vi "Export Origin - cDLTS.vi"(8 "Error In":errorcluster, 9 "Workspace":path, 10 "Session properties":T2, 11 "cDLTS measurement":T3={"Name"="", "Comment"="", "Time"=timestamp(0 s since 1904-01-01), "Folder"=path "", "DLTS properties"={"Tstart"=100.0, "Instant start"=FALSE, "Tstop"=350.0, "T rate"=0.016666666666666666, "Test signal"=0.1, "Test frequency"=100000.0, "Bandwidth"=0.0, "Averaging"=5.0, "Vbias"=-5.0, "Vpulse"=-1.0, "pulse length"=0.1, "Pulse 2"=FALSE, "Vpulse 2"=0.0, "pulse length 2"=0.0, "I range"=-2.0, "V range"=10.0, "Emission rate"=[10.0], "Sampling rate"=107000.0, "Acq. delay"=0.0}, "GUID"=""} {"DLTS properties"."V range" items=["10mV"=0.01, "100mV"=0.1, "1V"=1.0, "10V"=10.0]; "DLTS properties"."I range" items=["10mV"=0.01, "100mV"=0.1, "1V"=1.0, "10V"=10.0]}) -> (0 "Error Out":errorcluster)   [LabVIEW 2019]
doc: "Handles export of a DLTS measurement to an Origin project, displays a GUI window"
uses:
  Type defs/cDLTS measurement Type Def.ctl
  Type defs/DLTS properties Type Def.ctl
  Type defs/Session properties Type Def.ctl
  <vilib>/Utility/sysdir.llb/System Directory Type.ctl
panel:
  in  "Comment":T1(array[ring])=[enum."Emission rate"] caption="Parameters to be placed in comments"
  in  "Save and exit after export":bool
  in  "Export to current Origin instance":bool
  out "String":string
  in  "Path":path caption="Export file as:"
  in  "Export":bool
  in  "Cancel":bool
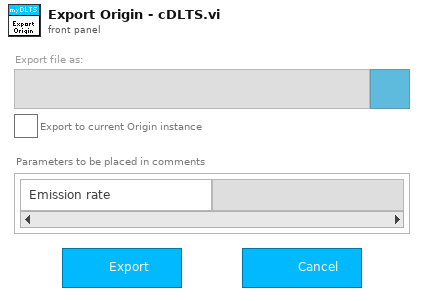
[diagram p1: front panel]
types:
  T1 = enum16{"", "Emission rate", "Temperature change rate", "Test signal", "Test frequency", "Bandwidth", "Averaging", "Bias voltage", "Pulse 1 voltage", "Pulse 1 length", "Pulse 2 voltage", "Pulse 2 length", "Current range", "Voltage range", "Sampling rate", "Acquisition delay"}[]
  T2 = typedef "Session properties Type Def.ctl" = cluster{"Session name":string, "Comment":string, "User":string, "Software version":dbl, "Created":timestamp, "Modified":timestamp, "Binary":bool, "GUID":string}
  T3 = typedef "cDLTS measurement Type Def.ctl" = cluster{"Name":string, "Comment":string, "Time":timestamp, "Folder":path, "DLTS properties":T4, "GUID":string}
  T4 = typedef "DLTS properties Type Def.ctl" = cluster{"Tstart":dbl[unit], "Instant start":bool, "Tstop":dbl[unit], "T rate":dbl[unit], "Test signal":dbl[unit], "Test frequency":dbl[unit], "Bandwidth":dbl[unit], "Averaging":dbl, "Vbias":dbl[unit], "Vpulse":dbl[unit], "pulse length":dbl[unit], "Pulse 2":bool, "Vpulse 2":dbl[unit], "pulse length 2":dbl[unit], "I range":dbl, "V range":dbl[unit], "Emission rate":dbl[unit][], "Sampling rate":dbl[unit], "Acq. delay":dbl[unit]}
  T5 = enum32{"existing file", "new file", "new or existing file", "existing dir", "new dir", "new or existing dir", "existing file (use LLBs)", "new file (use LLBs)", "new or existing file (use LLBs)", "new or existing file or directory (use LLBs)", "existing dir (use LLBs)", "new dir (use LLBs)", "new or existing dir (use LLBs)", "existing file or dir", "new file or dir", "new or existing file or dir", "existing file or dir (use LLBs)", "new file or dir (use LLBs)"}
  T6 = typedef "System Directory Type.ctl" = i32
  T7 = enum8{"Enabled", "Disabled", "Disabled and Grayed Out"}
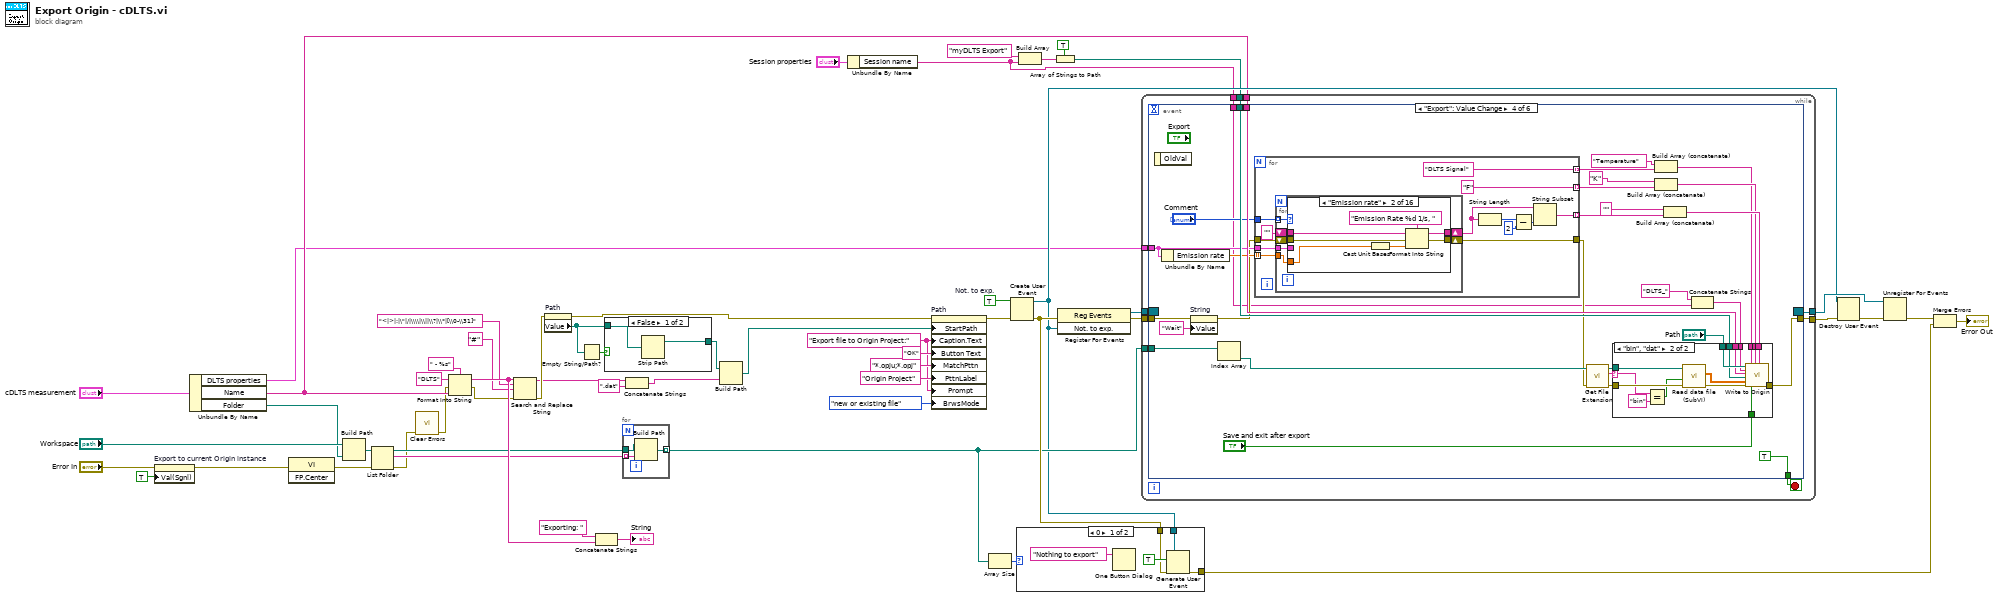
[diagram p0: block diagram]
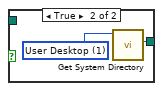
[diagram p2: hidden frame]
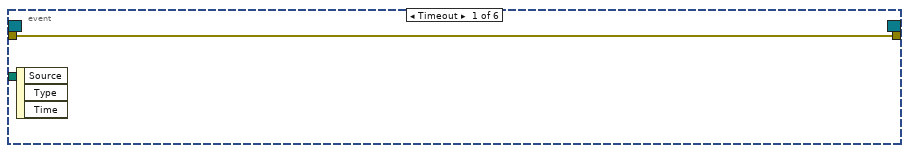
[diagram p4: hidden frame]
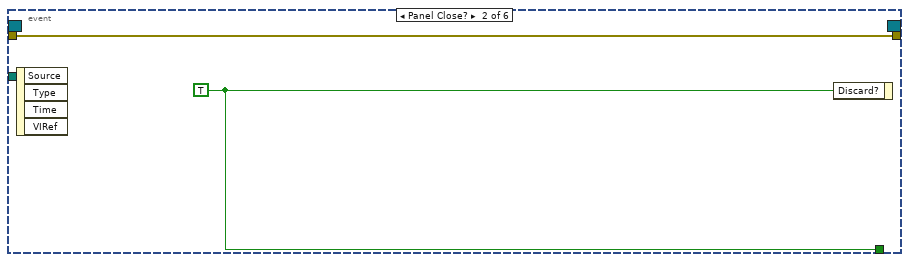
[diagram p5: hidden frame]
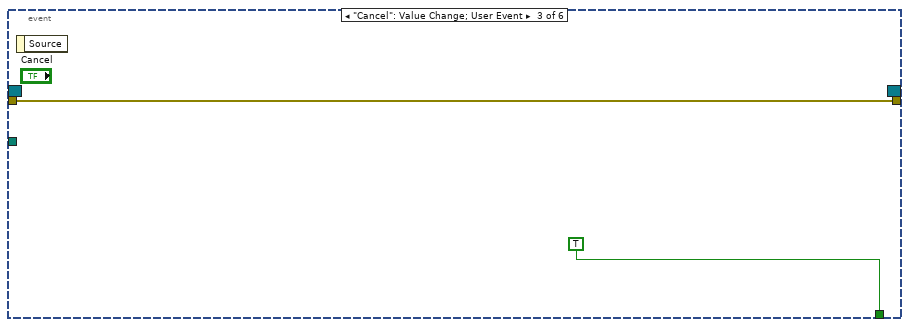
[diagram p6: hidden frame]
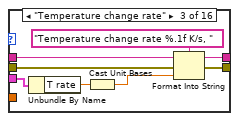
[diagram p8: hidden frame]
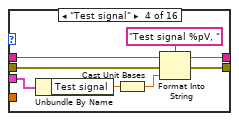
[diagram p9: hidden frame]
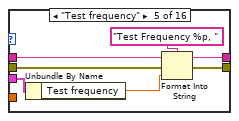
[diagram p10: hidden frame]
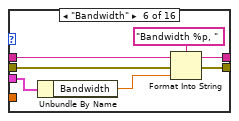
[diagram p11: hidden frame]
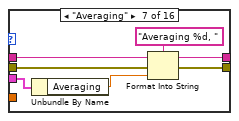
[diagram p12: hidden frame]
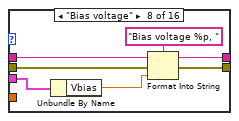
[diagram p13: hidden frame]
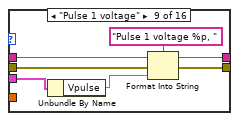
[diagram p14: hidden frame]
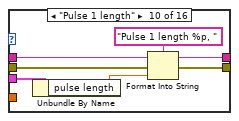
[diagram p15: hidden frame]
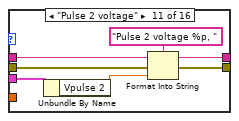
[diagram p16: hidden frame]
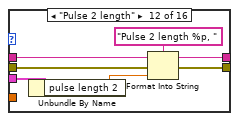
[diagram p17: hidden frame]
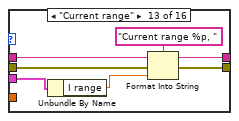
[diagram p18: hidden frame]
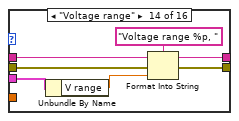
[diagram p19: hidden frame]
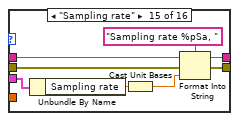
[diagram p20: hidden frame]
diagram:
  w27 = "Export file to Origin Project:"
  w54 = TRUE  # Not. to exp.
  n1 = property on="Export to current Origin instance" class="Bool (strict)"(error in="Error In", "Val(Sgnl)"=TRUE ("Value (Signaling)")) -> (error out=w6:errorcluster)  [unwired: 1 in, 1 out]
  n2 = Unbundle By Name("cDLTS measurement") -> ("DLTS properties"=w3:T4, "Name"=w14:string, "Folder"=w32:path)
  n3 = invoke class="VI" method="FP.Center"(error in=w6) -> (error out=w16:errorcluster)  [unwired: 2 in, 2 out]
  n4 = Build Path(base path="Workspace", name or relative path=w32) -> (appended path=w25:path)
  n5 = List Folder(path=w25, error in=w16) -> (path out=w24:path, filenames=w31:string[], error out=w20:errorcluster)  [unwired: 2 in, 1 out]
  n6 = call <vilib>:"Clear Errors.vi"("error in (no error)"=w20) -> ("error out"=w1:errorcluster)  [unwired: 5 in, 1 out]
  n7 = Format Into String(format string=" - %s", initial string="DLTS", error in=w1, w14) -> (resulting string=w43:string, error out=w19:errorcluster)
  n8 = Search and Replace String(input string=w43, search string="<|>|:|\"|/|\\\\|\\||\\?|\\*|[\\0-\\31]", replace string="#" ("replace string (\"\")"), error in=w19) -> (result string=w18:string, error out=w21:errorcluster)  [unwired: 4 in, 2 out]
  n9 = property on="Path" class="Path"(error in=w21) -> (error out=w33:errorcluster, "Value"=w39:path)  [unwired: 1 in, 1 out]
  n10 = Empty String/Path?(string/path=w39) -> (empty?=w40:bool)
  n11 = Concatenate Strings("Exporting: " ("string"), w43) -> (→"String":string)
  n12 = case shown="False" w40 {
    tunnel: w39 -> [w58 _]
    tunnel: [w57 w59] -> w35
    frame False {
      n13 = Strip Path(path=w58) -> (stripped path=w57:path)  [unwired: 1 out]
    }
    frame True {
      w60 = T6 1 items=["User Home"=0, "User Desktop"=1, "User Documents"=2, "User Application Data"=3, "User Preferences"=4, "User Temporary"=5, "Public Documents"=6, "Public Application Data"=7, "Public Preferences"=8, "Public Cache"=13, "System Core Libraries"=9, "System Installed Libraries"=10, "Application Files"=11, "Boot Volume Root"=12] ("system directory type")
      n14 = call <vilib>:"Get System Directory.vi"("system directory type"=w60) -> ("system directory"=w59:path)  [unwired: 10 in]
    }
  }
  n15 = for {
    tunnel: w24 -> [w63]
    tunnel: [w62] -> w49 mode=indexing
    tunnel: w31 -> [w61] mode=indexing
    n16 = Build Path(base path=w63, name or relative path=w61) -> (appended path=w62:path)
  }
  n17 = Concatenate Strings(w18, ".dat" ("string")) -> (w22:string)
  n18 = Build Path(base path=w35, name or relative path=w22) -> (appended path=w34:path)
  n19 = Unbundle By Name("Session properties") -> ("Session name"=w2:string)
  n20 = property on="Path" class="Path"(error in=w33, "StartPath"=w34, "Caption.Text"=w27, "Button Text"="OK", "MatchPttn"="*.opju;*.opj", "PttnLabel"="Origin Project", "Prompt"=w27, "BrwsMode"=T5."new or existing file" ("Browse Options:Selection Mode")) -> (error out=w51:errorcluster)  [unwired: 1 in, 1 out]
  n21 = Array Size(array=w49) -> (size(s)=w55:i32)
  n22 = Create User Event(user event datatype=w54, error in=w51) -> (user event=w15:refnum<user-event>, error out=w50:errorcluster)
  n23 = case shown="0" w55 {
    tunnel: w15 -> [w67 _]
    tunnel: w50 -> [w65 w69]
    tunnel: [w64 w69] -> w44
    frame 0 {
      n24 = One Button Dialog(message="Nothing to export") -> ()  [unwired: 1 in, 1 out]
      n25 = Generate User Event(user event=w67, event data cluster=TRUE ("event data"), error in=w65) -> (error out=w64:errorcluster)  [unwired: 1 in, 1 out]
    }
    frame Default {
    }
  }
  n26 = Build Array("myDLTS Export" ("element"), w2) -> (w10:string[])
  n27 = Array of Strings to Path(0:w10, 1:TRUE ("relative")) -> (2:w9:path)
  n28 = register-events(error in=w50, w15) -> (reference out=w52:refnum<event-registration>, error out=w53:errorcluster)  [unwired: 1 in]
  n29 = while {
    tunnel: w53 -> [w79]
    tunnel: w49 -> [w77]
    tunnel: w52 -> [w76]
    tunnel: [w75] -> w47
    tunnel: w14 -> [w74]
    tunnel: w9 -> [w73]
    tunnel: [w72] -> w8
    tunnel: w3 -> [w71]
    tunnel: w2 -> [w70]
    stop <- w78 stop-if-true
    n30 = event shown="[3] \"Export\": Value Change" {
      selector: w76 -> [_ _ _ _ _ _]
      dyn-events: [_ _ _ _ _ _] -> w75
      timeout: _ -> [_ _ _ _ _ _]
      tunnel: w79 -> [w80 w81 w83 w109 w269 w276]
      tunnel: [w80 w81 w83 w112 w262 w271] -> w72
      tunnel: [_ w82 TRUE ("Discard?") TRUE _ _] -> w78
      tunnel: w77 -> [_ _ _ w114 _ _]
      tunnel: w74 -> [_ _ _ w107 _ _]
      tunnel: w73 -> [_ _ _ w106 _ _]
      tunnel: w71 -> [_ _ _ w90 _ _]
      tunnel: w70 -> [_ _ _ w85 _ _]
      event Timeout {
        n31 = event-data() -> ()  [unwired: 1 in, 3 out]
      }
      event Panel Close? {
        w82 = TRUE ("Discard?")
        n32 = event-data() -> ()  [unwired: 1 in, 4 out]
        n33 = event-data("Discard?"=w82) -> ()  [unwired: 1 in, 1 out]
      }
      event "Cancel": Value Change; User Event {
        n34 = event-data() -> ()  [unwired: 1 in, 1 out]
      }
      event "Export": Value Change {
        n35 = event-data() -> ()  [unwired: 1 in, 1 out]
        n36 = Unbundle By Name(w90) -> ("Emission rate"=w91:dbl[unit][])
        n37 = property on="String" class="Str"(error in=w109, "Value"="Wait" ("String")) -> (error out=w89:errorcluster)  [unwired: 1 in, 1 out]
        n38 = Index Array(array=w114) -> (element=w102:path)  [unwired: 1 in]
        n39 = for {
          tunnel: w90 -> [w123]
          tunnel: [w119] -> w98 mode=indexing
          tunnel: ["DLTS Signal"] -> w100 mode=indexing
          tunnel: ["F"] -> w99 mode=indexing
          tunnel: "Comment" -> [w125]
          tunnel: w91 -> [w122] mode=indexing
          tunnel: w89 -> [w121]
          tunnel: [w120] -> w88
          n40 = for {
            tunnel: w125 -> [w134] mode=indexing
            tunnel: w123 -> [w133]
            shift-right: [w132] -> w120
            shift-left: w121 -> [w131]
            shift-right: [w130] -> w118
            shift-left: "" -> [w129]
            tunnel: w122 -> [w128]
            n41 = case shown="\"Emission rate\"" w134 {
              tunnel: w133 -> [_ _ w147 w153 w160 w167 w174 w181 w188 w195 w202 w209 w216 w223 w231 w238]
              tunnel: w128 -> [_ w142 _ _ _ _ _ _ _ _ _ _ _ _ _ _]
              tunnel: [w135 w141 w151 w157 w162 w171 w178 w185 w192 w199 w206 w213 w220 w227 w235 w242] -> w132
              tunnel: w131 -> [w135 w140 w149 w155 w164 w169 w176 w182 w189 w196 w203 w210 w217 w224 w232 w239]
              tunnel: [w136 w139 w150 w156 w161 w170 w177 w184 w191 w198 w205 w212 w219 w226 w234 w241] -> w130
              tunnel: w129 -> [w136 w138 w148 w154 w163 w168 w175 w183 w190 w197 w204 w211 w218 w225 w233 w240]
              frame "", Default {
              }
              frame "Emission rate" {
                n42 = Cast Unit Bases(0:w142) -> (2:w137:dbl)  [unwired: 1 in]
                n43 = Format Into String(format string="Emission Rate %d 1/s, ", initial string=w138, error in=w140, w137) -> (resulting string=w139:string, error out=w141:errorcluster)
              }
              frame "Temperature change rate" {
                n44 = Unbundle By Name(w147) -> ("T rate"=w146:dbl[unit])
                n45 = Cast Unit Bases(0:w146) -> (2:w144:dbl)  [unwired: 1 in]
                n46 = Format Into String(format string="Temperature change rate %.1f K/s, ", initial string=w148, error in=w149, w144) -> (resulting string=w150:string, error out=w151:errorcluster)
              }
              frame "Test signal" {
                n47 = Unbundle By Name(w153) -> ("Test signal"=w158:dbl[unit])
                n48 = Cast Unit Bases(0:w158) -> (2:w152:dbl)  [unwired: 1 in]
                n49 = Format Into String(format string="Test signal %pV, ", initial string=w154, error in=w155, w152) -> (resulting string=w156:string, error out=w157:errorcluster)
              }
              frame "Test frequency" {
                n50 = Unbundle By Name(w160) -> ("Test frequency"=w165:dbl[unit])
                n51 = Format Into String(format string="Test Frequency %p, ", initial string=w163, error in=w164, w165) -> (resulting string=w161:string, error out=w162:errorcluster)
              }
              frame "Bandwidth" {
                n52 = Unbundle By Name(w167) -> ("Bandwidth"=w172:dbl[unit])
                n53 = Format Into String(format string="Bandwidth %p, ", initial string=w168, error in=w169, w172) -> (resulting string=w170:string, error out=w171:errorcluster)
              }
              frame "Averaging" {
                n54 = Unbundle By Name(w174) -> ("Averaging"=w179:dbl)
                n55 = Format Into String(format string="Averaging %d, ", initial string=w175, error in=w176, w179) -> (resulting string=w177:string, error out=w178:errorcluster)
              }
              frame "Bias voltage" {
                n56 = Unbundle By Name(w181) -> ("Vbias"=w186:dbl[unit])
                n57 = Format Into String(format string="Bias voltage %p, ", initial string=w183, error in=w182, w186) -> (resulting string=w184:string, error out=w185:errorcluster)
              }
              frame "Pulse 1 voltage" {
                n58 = Unbundle By Name(w188) -> ("Vpulse"=w193:dbl[unit])
                n59 = Format Into String(format string="Pulse 1 voltage %p, ", initial string=w190, error in=w189, w193) -> (resulting string=w191:string, error out=w192:errorcluster)
              }
              frame "Pulse 1 length" {
                n60 = Unbundle By Name(w195) -> ("pulse length"=w200:dbl[unit])
                n61 = Format Into String(format string="Pulse 1 length %p, ", initial string=w197, error in=w196, w200) -> (resulting string=w198:string, error out=w199:errorcluster)
              }
              frame "Pulse 2 voltage" {
                n62 = Unbundle By Name(w202) -> ("Vpulse 2"=w207:dbl[unit])
                n63 = Format Into String(format string="Pulse 2 voltage %p, ", initial string=w204, error in=w203, w207) -> (resulting string=w205:string, error out=w206:errorcluster)
              }
              frame "Pulse 2 length" {
                n64 = Unbundle By Name(w209) -> ("pulse length 2"=w214:dbl[unit])
                n65 = Format Into String(format string="Pulse 2 length %p, ", initial string=w211, error in=w210, w214) -> (resulting string=w212:string, error out=w213:errorcluster)
              }
              frame "Current range" {
                n66 = Unbundle By Name(w216) -> ("I range"=w221:dbl)
                n67 = Format Into String(format string="Current range %p, ", initial string=w218, error in=w217, w221) -> (resulting string=w219:string, error out=w220:errorcluster)
              }
              frame "Voltage range" {
                n68 = Unbundle By Name(w223) -> ("V range"=w228:dbl[unit])
                n69 = Format Into String(format string="Voltage range %p, ", initial string=w225, error in=w224, w228) -> (resulting string=w226:string, error out=w227:errorcluster)
              }
              frame "Sampling rate" {
                n70 = Unbundle By Name(w231) -> ("Sampling rate"=w236:dbl[unit])
                n71 = Cast Unit Bases(0:w236) -> (2:w230:dbl)  [unwired: 1 in]
                n72 = Format Into String(format string="Sampling rate %pSa, ", initial string=w233, error in=w232, w230) -> (resulting string=w234:string, error out=w235:errorcluster)
              }
              frame "Acquisition delay" {
                n73 = Unbundle By Name(w238) -> ("Sampling rate"=w243:dbl[unit])
                n74 = Format Into String(format string="Acquisition delay %p, ", initial string=w240, error in=w239, w243) -> (resulting string=w241:string, error out=w242:errorcluster)
              }
            }
          }
          n75 = String Length(string=w118) -> (length=w117:i32)
          n76 = Subtract(x=w117, y=2) -> (x-y=w116:i32)
          n77 = String Subset(string=w118, length (rest)=w116) -> (substring=w119:string)  [unwired: 1 in]
        }
        n78 = call <vilib>:"Get File Extension.vi"("error in (no error)"=w88, "file"=w102) -> ("error out"=w104:errorcluster, "lowercase file extension"=w103:string, "dup file"=w105:path)  [unwired: 5 in, 2 out]
        n79 = Build Array (concatenate)("Temperature", w100) -> (w92:string[])
        n80 = Build Array (concatenate)("K", w99) -> (w93:string[])
        n81 = Build Array (concatenate)("", w98) -> (w94:string[])
        n82 = Concatenate Strings("DLTS_" ("Book name"), w85) -> (w86:string)
        n83 = case shown="\"bin\", \"dat\"" w103 {
          selector: w103 -> [_ w246]
          tunnel: w105 -> [_ w260]
          tunnel: w104 -> [w245 w259]
          tunnel: "Path" -> [_ w255]
          tunnel: w92 -> [_ w254]
          tunnel: w93 -> [_ w253]
          tunnel: w94 -> [_ w252]
          tunnel: [w245 w251] -> w112
          tunnel: "Save and exit after export" -> [_ w250]
          tunnel: w86 -> [_ w249]
          tunnel: w107 -> [_ w248]
          tunnel: w106 -> [_ w247]
          frame "False", Default {
          }
          frame "bin", "dat" {
            n84 = Equal?(x=w246, y="bin") -> (x = y?=w258:bool)
            n85 = call "Read data file (SubVI).vi"("error in"=w259, "Binary"=w258, "file path in"=w260) -> ("error out"=w256:errorcluster, "2D data"=w257:dbl[][])  [unwired: 6 in, 1 out]
            n86 = call "Write to Origin.vi"("Origin Project Path"=w255, "Book name"=w249, "Sheet name"=w248, "Folder name"=w247, "Data"=w257, "error in (no error)"=w256, "Column name"=w254, "Save and exit"=w250, "Column unit"=w253, "Column comment"=w252) -> ("error out"=w251:errorcluster)  [unwired: 9 in]
          }
        }
      }
      event "Export to current Origin instance": Value Change {
        n87 = event-data() -> ("NewVal"=w264:bool)  [unwired: 1 in]
        n88 = Select(t=T7."Disabled and Grayed Out" ("Disabled"), s=w264, f=T7."Enabled" ("Disabled")) -> (s? t:f=w265:T7)
        n89 = property on="Path" class="Path"(error in=w269, "Val(Sgnl)"=path "" ("Value (Signaling)"), "DisabledEnum"=w265) -> (error out=w268:errorcluster)  [unwired: 1 in, 1 out]
        n90 = Not(x=w264) -> (.not. x?=w263:bool)
        n91 = property on="Save and exit after export" class="Bool (strict)"(error in=w268, "Visible"=w263) -> (error out=w262:errorcluster)  [unwired: 1 in, 1 out]
      }
      event "Path": Value Change {
        n92 = event-data() -> ("NewVal"=w280:path)  [unwired: 1 in]
        n93 = Path Type(1:w280) -> (0:w279:i16)
        n94 = Equal To 0?(x=w279) -> (x = 0?=w277:bool)
        n95 = Or(x=w277, y="Export to current Origin instance") -> (x .or. y?=w275:bool)
        n96 = Select(t=T7."Enabled" ("Disabled"), s=w275, f=T7."Disabled and Grayed Out") -> (s? t:f=w274:T7)
        n97 = property on="Export" class="Bool"(error in=w276, "DisabledEnum"=w274) -> (error out=w271:errorcluster)  [unwired: 1 in, 1 out]
      }
    }
  }
  n98 = Destroy User Event(user event=w15, error in=w8) -> (error out=w48:errorcluster)
  n99 = Unregister For Events(event registration refnum=w47, error in=w48) -> (error out=w46:errorcluster)
  n100 = Merge Errors(w46, w44) -> (→"Error Out":errorcluster)
